vi "Decompose LabVIEW Object - Child - Private Data Cluster Count.vi"() -> ()   [LabVIEW 2017, in "Composition.Tests.lvlib"]
uses:
  Composition.Tests.lvlib
  Classes/Child/Child.lvclass
  Composition/Composition.lvlib
  <vilib>/addons/_JKI Toolkits/Caraya/classes/Assert/Assert.lvclass
  <vilib>/addons/_JKI Toolkits/Caraya/classes/Test/Test.lvclass
panel:
  out "error out":errorcluster
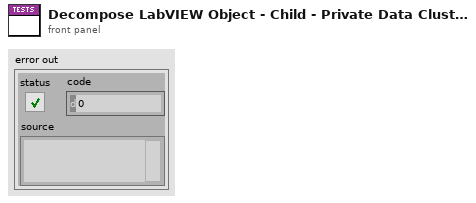
[diagram p1: front panel]
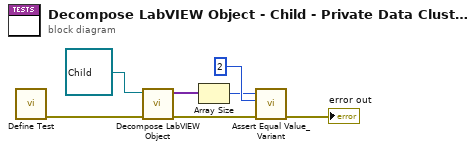
[diagram p0: block diagram]
diagram:
  n1 = call <vilib>:"Define Test.vi"() -> ("error out"=w2:errorcluster)  [unwired: 11 in]
  n2 = call "Decompose LabVIEW Object.vi"("error in (no error)"=w2, "LabVIEW Object"=refnum<class "Child.lvclass"> refnum ("Reflection.Tests.lvlib:Child.lvclass")) -> ("error out"=w6:errorcluster, "Private Data Clusters"=w4:variant[])  [unwired: 6 in, 2 out]
  n3 = Array Size(array=w4) -> (size(s)=w1:i32)
  n4 = call <vilib>:"Assert Equal Value_Variant.vi"("error in (no error)"=w6, "Y"=2 ("Expected"), "X"=w1) -> ("error out"=→"error out":errorcluster)  [unwired: 8 in]
